vi "Relay Experiment.vi"() -> ()   [LabVIEW 2020]
uses:
  <vilib>/Analysis/1siggen.llb/Ramp Pattern by Samples.vi
  <vilib>/DAQmx/write.llb/DAQmx Write (Analog 1D Wfm NChan NSamp).vi
  <vilib>/DAQmx/create/channels.llb/DAQmx Create Channel (AO-Voltage-Basic).vi
  <vilib>/Waveform/WDTOps.llb/WDT Append Waveforms DBL.vi
  <vilib>/Waveform/WDTOps.llb/WDT Number of Waveform Samples DBL.vi
  <vilib>/DAQmx/configure/timing.llb/DAQmx Timing (Sample Clock).vi
  <vilib>/DAQmx/miscellaneous.llb/DAQmx Fill In Error Info.vi
  <vilib>/DAQmx/configure/timing.llb/DAQmx Timing (Use Waveform).vi
  <vilib>/measure/NI_MABase.lvlib
  <vilib>/measure/NI_MAPro.lvlib
  <vilib>/Analysis/NI_AALBase.lvlib
panel:
  in  "AC Source\nGain":dbl=5.0
  out "DC On":bool=TRUE
  in  "Continue AC Waveform":bool=TRUE
  out "AC On":bool
  in  "Waveform Type":u16(ring) items=["Sine Wave", "Triangle Wave", "Square Wave", "Sawtooth Wave"]
  out "DC Waveform Graph":waveform(dbl)(graph)
  out "AC Sampling\nFrequency (Hz)":i64
  in  "AC  Waveform\nFrequency (Hz)":i64=20000 step=1
  out "DC Total\nTime (s)":dbl
  in  "DC Recharge\nRamp Time":dbl
  in  "AC  Waveform\nAmplitude\n(Vpp/mApp)":dbl
  out "DC Recharge\nTime (s)":dbl
  out "DC Pulse\nCharge (mC)":dbl
  in  "DC Recharge\nAmplitude (mA)":dbl
  in  "DC Pulse\nAmplitude (-mA)":dbl
  in  "DC Pulse\nTime (s)":dbl
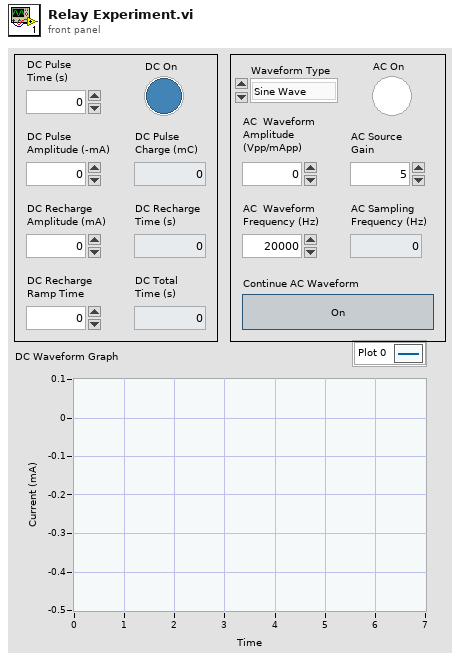
[diagram p1: front panel]
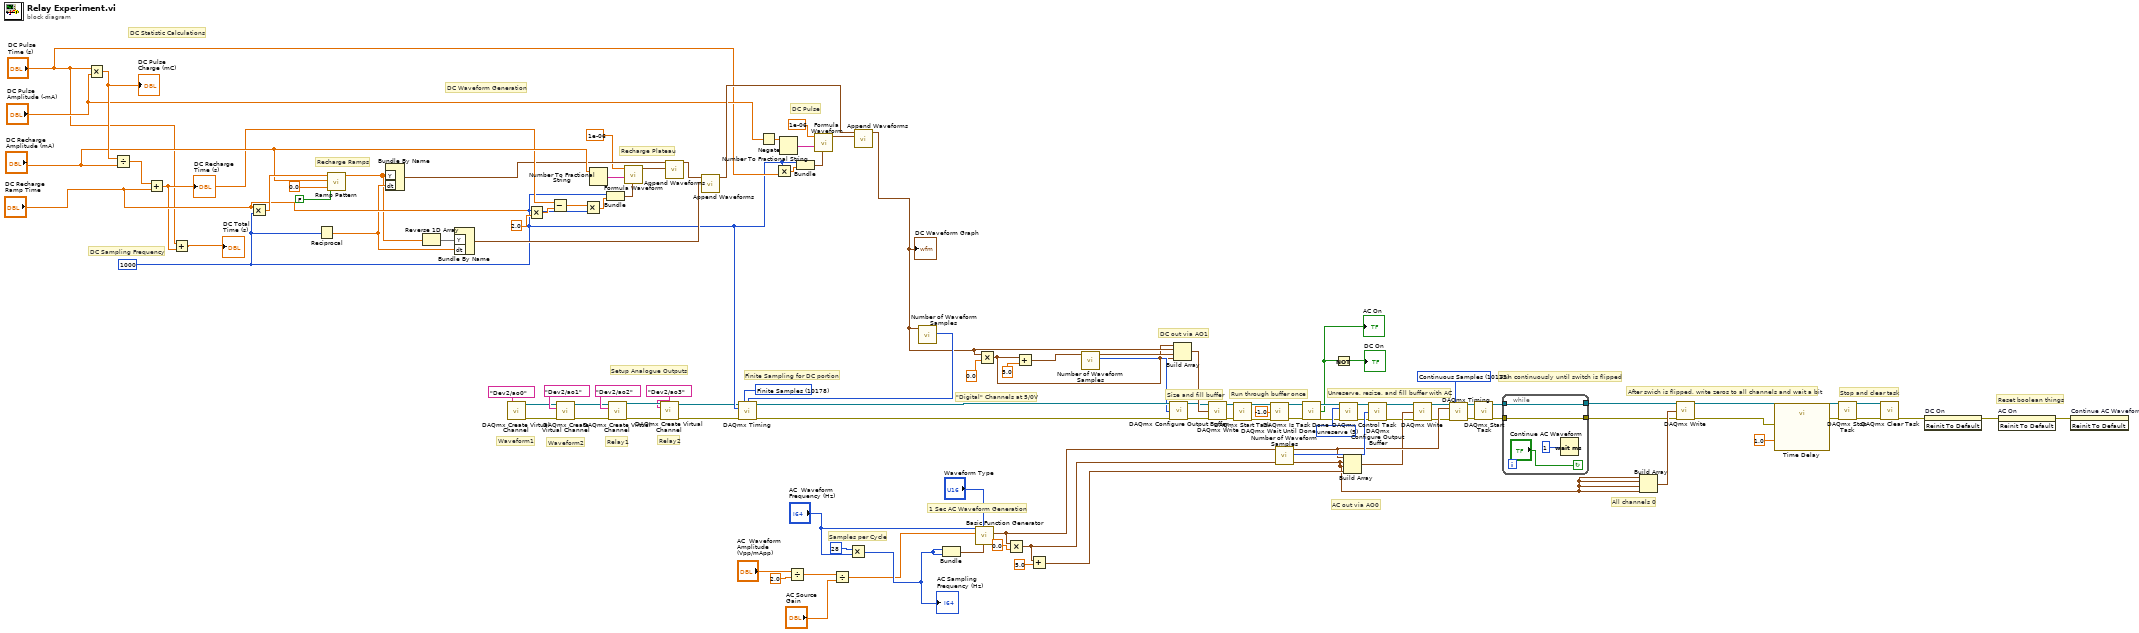
[diagram p0: block diagram]
diagram:
  w39 = 5 items=["verify"=2, "reserve"=4, "commit"=3, "unreserve"=5, "abort"=6] ("action")
  w44 = 10123 items=["Finite Samples"=10178, "Continuous Samples"=10123, "Hardware Timed Single Point"=12522] ("sample mode")
  w71 = 1000
  w67 = 10178 items=["Finite Samples"=10178, "Continuous Samples"=10123, "Hardware Timed Single Point"=12522] ("sample mode")
  # "AC out via AO0"
  # "DC out via AO1"
  # "Relay2"
  # "Relay1"
  # "Waveform2"
  # "Waveform1"
  # "Reset boolean things"
  # "Stop and clear task"
  # "All channels 0"
  # "After swich is flipped, write zeros to all channels and wait a bit"
  # "Run continuously until switch is flipped"
  # "Unreserve, resize, and fill buffer with AC"
  # "Run through buffer once"
  # "Size and fill buffer"
  # "\"Digital\" Channels at 5/0V"
  # "Finite Sampling for DC portion"
  # "DC Sampling Frequency"
  # "Setup Analogue Outputs"
  # "Samples per Cycle"
  # "1 Sec AC Waveform Generation"
  # "DC Pulse"
  # "Recharge Plateau"
  # "Recharge Ramps"
  # "DC Waveform Generation"
  # "DC Statistic Calculations"
  n1 = Multiply(x="DC Pulse\nTime (s)", y="DC Pulse\nAmplitude (-mA)") -> (x*y=w112:dbl)
  "DC Pulse\nCharge (mC)" <- w112
  n2 = Divide(x=w112, y="DC Recharge\nAmplitude (mA)") -> (x/y=w111:dbl)
  n3 = Add(x=w111, y="DC Recharge\nRamp Time") -> (x+y=w101:dbl)
  "DC Recharge\nTime (s)" <- w101
  n4 = Add(x="DC Pulse\nTime (s)", y=w101) -> (x+y=→"DC Total\nTime (s)":dbl)
  n5 = Multiply(x="DC Recharge\nRamp Time", y=w71) -> (x*y=w108:dbl)
  n6 = Reciprocal(x=w71) -> (1/x=w95:dbl)
  n7 = call-poly <vilib>:"Ramp Pattern.vi"("exclude end?"=FALSE, "start"=0.0, "end"="DC Recharge\nAmplitude (mA)", "samples"=w108) -> ("Ramp Pattern"=w93:dbl[])  [unwired: 6 in, 1 out]
  n8 = Bundle By Name("Y"=w93, "dt"=w95) -> (w98:waveform(dbl))  [unwired: 1 in]
  n9 = Reverse 1D Array(array=w93) -> (reversed array=w94:dbl[])
  n10 = Bundle By Name("Y"=w94, "dt"=w95) -> (w91:waveform(dbl))  [unwired: 1 in]
  n11 = call-poly <vilib>:"DAQmx Create Virtual Channel.vi"("physical channels"=tag "Dev2/ao0") -> ("task out"=w77:refnum<k21>, "error out"=w70:errorcluster)  [unwired: 13 in]
  n12 = Multiply(x="DC Recharge\nRamp Time", y=2.0) -> (x*y=w105:dbl)
  n13 = Subtract(x=w101, y=w105) -> (x-y=w99:dbl)
  n14 = call-poly <vilib>:"DAQmx Create Virtual Channel.vi"("task in"=w77, "physical channels"=tag "Dev2/ao1", "error in"=w70) -> ("task out"=w61:refnum<k21>, "error out"=w60:errorcluster)  [unwired: 11 in]
  n15 = Multiply(x=w99, y=w71) -> (x*y=w100:dbl)
  n16 = Number To Fractional String(number="DC Recharge\nAmplitude (mA)") -> (F-format string=w107:string)  [unwired: 3 in]
  n17 = Bundle(w71, w100) -> (w102:cluster{i32, dbl})  [unwired: 1 in]
  n18 = call-poly <vilib>:"DAQmx Create Virtual Channel.vi"("task in"=w61, "physical channels"=tag "Dev2/ao2", "error in"=w60) -> ("task out"=w30:refnum<k21>, "error out"=w29:errorcluster)  [unwired: 11 in]
  n19 = call <vilib>:"Formula Waveform.vi"("sampling info"=w102, "formula"=w107, "frequency"=1e-06) -> ("signal out"=w97:waveform(dbl))  [unwired: 7 in, 1 out]
  n20 = call-poly <vilib>:"DAQmx Create Virtual Channel.vi"("task in"=w30, "physical channels"=tag "Dev2/ao3", "error in"=w29) -> ("task out"=w31:refnum<k21>, "error out"=w32:errorcluster)  [unwired: 11 in]
  n21 = call-poly <vilib>:"Append Waveforms.vi"("waveform B"=w97, "waveform A"=w98) -> ("waveform out"=w92:waveform(dbl))  [unwired: 8 in, 1 out]
  n22 = call-poly <vilib>:"Append Waveforms.vi"("waveform B"=w91, "waveform A"=w92) -> ("waveform out"=w87:waveform(dbl))  [unwired: 8 in, 1 out]
  n23 = Negate(x="DC Pulse\nAmplitude (-mA)") -> (-x=w86:dbl)
  n24 = Multiply(x=w71, y="DC Pulse\nTime (s)") -> (x*y=w89:dbl)
  n25 = Number To Fractional String(number=w86) -> (F-format string=w90:string)  [unwired: 3 in]
  n26 = Divide(x="AC  Waveform\nAmplitude\n(Vpp/mApp)", y=2.0) -> (x/y=w2:dbl)
  n27 = Bundle(w71, w89) -> (w83:cluster{i32, dbl})  [unwired: 1 in]
  n28 = call <vilib>:"Formula Waveform.vi"("sampling info"=w83, "formula"=w90, "frequency"=1e-06) -> ("signal out"=w88:waveform(dbl))  [unwired: 7 in, 1 out]
  n29 = Divide(x=w2, y="AC Source\nGain") -> (x/y=w3:dbl)
  n30 = Multiply(x=i64 28, y="AC  Waveform\nFrequency (Hz)") -> (x*y=w52:i64)
  "AC Sampling\nFrequency (Hz)" <- w52
  n31 = call-poly <vilib>:"Append Waveforms.vi"("waveform B"=w88, "waveform A"=w87) -> ("waveform out"=w45:waveform(dbl))  [unwired: 8 in, 1 out]
  "DC Waveform Graph" <- w45
  n32 = call-poly <vilib>:"Number of Waveform Samples.vi"("waveform in"=w45) -> ("number of samples"=w54:i32)  [unwired: 8 in, 2 out]
  n33 = call-poly <vilib>:"DAQmx Timing.vi"("task/channels in"=w31, "sample mode"=w67, "samples per channel"=w54, "rate"=w71, "error in"=w32) -> ("task out"=w72:refnum<k21>, "error out"=w69:errorcluster)  [unwired: 9 in]
  n34 = Bundle(w52, w52) -> (w84:cluster{i64, i64})  [unwired: 1 in]
  n35 = call <vilib>:"Basic Function Generator.vi"("sampling info"=w84, "signal type"="Waveform Type", "amplitude"=w3, "frequency"="AC  Waveform\nFrequency (Hz)") -> ("signal out"=w46:waveform(dbl))  [unwired: 5 in, 2 out]
  n36 = Multiply(x=w45, y=0.0) -> (x*y=w4:waveform(dbl))
  n37 = Multiply(x=w46, y=0.0) -> (x*y=w5:waveform(dbl))
  n38 = Add(x=w4, y=5.0) -> (x+y=w8:waveform(dbl))
  n39 = Add(x=w5, y=5.0) -> (x+y=w6:waveform(dbl))
  n40 = call-poly <vilib>:"Number of Waveform Samples.vi"("waveform in"=w8) -> ("number of samples"=w53:i32, "waveform out"=w7:waveform(dbl))  [unwired: 8 in, 1 out]
  n41 = call <vilib>:"DAQmx Configure Output Buffer.vi"("task/channels in"=w72, "buffer size (in samples per channel)"=w53, "error in"=w69) -> ("task out"=w63:refnum<k21>, "error out"=w34:errorcluster)  [unwired: 11 in]
  n42 = Build Array(w4, w45, w7, w4) -> (w73:waveform(dbl)[])
  n43 = call-poly <vilib>:"DAQmx Write.vi"("task/channels in"=w63, "data"=w73, "error in"=w34) -> ("task out"=w64:refnum<k21>, "error out"=w33:errorcluster)  [unwired: 10 in, 1 out]
  n44 = call <vilib>:"DAQmx Start Task.vi"("task/channels in"=w64, "error in"=w33) -> ("task out"=w65:refnum<k21>, "error out"=w66:errorcluster)  [unwired: 12 in]
  n45 = call <vilib>:"DAQmx Wait Until Done.vi"("task/channels in"=w65, "timeout (sec)"=-1.0, "error in"=w66) -> ("task out"=w25:refnum<k21>, "error out"=w24:errorcluster)  [unwired: 11 in]
  n46 = call-poly <vilib>:"Number of Waveform Samples.vi"("waveform in"=w46) -> ("number of samples"=w49:i32, "waveform out"=w48:waveform(dbl))  [unwired: 8 in, 1 out]
  n47 = call <vilib>:"DAQmx Is Task Done.vi"("task/channels in"=w25, "error in"=w24) -> ("task out"=w23:refnum<k21>, "task done?"=w21:bool, "error out"=w22:errorcluster)  [unwired: 11 in]
  "AC On" <- w21
  n48 = Not(x=w21) -> (.not. x?=→"DC On":bool)
  n49 = call <vilib>:"DAQmx Control Task.vi"("task/channels in"=w23, "action"=w39, "error in"=w22) -> ("task out"=w41:refnum<k21>, "error out"=w40:errorcluster)  [unwired: 11 in]
  n50 = Build Array(w48, w5, w5, w6) -> (w47:waveform(dbl)[])
  n51 = call <vilib>:"DAQmx Configure Output Buffer.vi"("task/channels in"=w41, "buffer size (in samples per channel)"=w49, "error in"=w40) -> ("task out"=w36:refnum<k21>, "error out"=w35:errorcluster)  [unwired: 11 in]
  n52 = call-poly <vilib>:"DAQmx Write.vi"("task/channels in"=w36, "data"=w47, "error in"=w35) -> ("task out"=w37:refnum<k21>, "error out"=w38:errorcluster)  [unwired: 10 in, 1 out]
  n53 = call-poly <vilib>:"DAQmx Timing.vi"("task/channels in"=w37, "sample mode"=w44, "waveform"=w48, "error in"=w38) -> ("task out"=w43:refnum<k21>, "error out"=w42:errorcluster)  [unwired: 10 in]
  n54 = call <vilib>:"DAQmx Start Task.vi"("task/channels in"=w43, "error in"=w42) -> ("task out"=w16:refnum<k21>, "error out"=w15:errorcluster)  [unwired: 12 in]
  n55 = while {
    tunnel: w16 -> [w113]
    tunnel: w15 -> [w114]
    tunnel: [w113] -> w14
    tunnel: [w114] -> w13
    stop <- "Continue AC Waveform" continue-if-true
    n56 = Wait (ms)(milliseconds to wait=u32 1) -> ()  [unwired: 1 out]
  }
  n57 = Build Array(w5, w5, w5, w5) -> (w26:waveform(dbl)[])
  n58 = call-poly <vilib>:"DAQmx Write.vi"("task/channels in"=w14, "data"=w26, "error in"=w13) -> ("task out"=w10:refnum<k21>, "error out"=w9:errorcluster)  [unwired: 10 in, 1 out]
  n59 = call "Time Delay"("error in (no error)"=w9, "Delay Time (s)"=1.0) -> ("error out"=w12:errorcluster)  [unwired: 9 in]
  n60 = call <vilib>:"DAQmx Stop Task.vi"("task/channels in"=w10, "error in"=w12) -> ("task out"=w57:refnum<k21>, "error out"=w56:errorcluster)  [unwired: 12 in]
  n61 = call <vilib>:"DAQmx Clear Task.vi"("task in"=w57, "error in"=w56) -> ("error out"=w19:errorcluster)  [unwired: 13 in]
  n62 = invoke on="DC On" class="Bool (strict)" method="Reinit To Default"(error in=w19) -> (error out=w18:errorcluster)  [unwired: 2 in, 2 out]
  n63 = invoke on="AC On" class="Bool (strict)" method="Reinit To Default"(error in=w18) -> (error out=w17:errorcluster)  [unwired: 2 in, 2 out]
  n64 = invoke on="Continue AC Waveform" class="Bool (strict)" method="Reinit To Default"(error in=w17) -> ()  [unwired: 2 in, 3 out]
